vi "Set (Str).vi"(6 "ISOBUS address":T3=-1 caption="ISOBUS address (-1)", 8 "error in":errorcluster, 9 "Command Value (Str)":string, 10 "SCPI Message(s)":string[](array[string]), 11 "Mercury Reference In":T4) -> (0 "error out":errorcluster, 2 "Response":T1, 3 "Mercury Reference Out":T4, 4 "Valid?":T2)   [LabVIEW 2019]
doc: "Write the selected value as a string to the specified command on the remote instrument."
uses:
  Public/Controls/Mercury Reference.ctl
  Public/Controls/Comms Transport Layer.ctl
  Private/Controls/Query Dynamic Reference.ctl
  Public/Controls/ISOBus Address.ctl
  Public/Controls/Is Valid LED.ctl
  Public/Controls/Response String.ctl
  Mercury iXX.lvlib
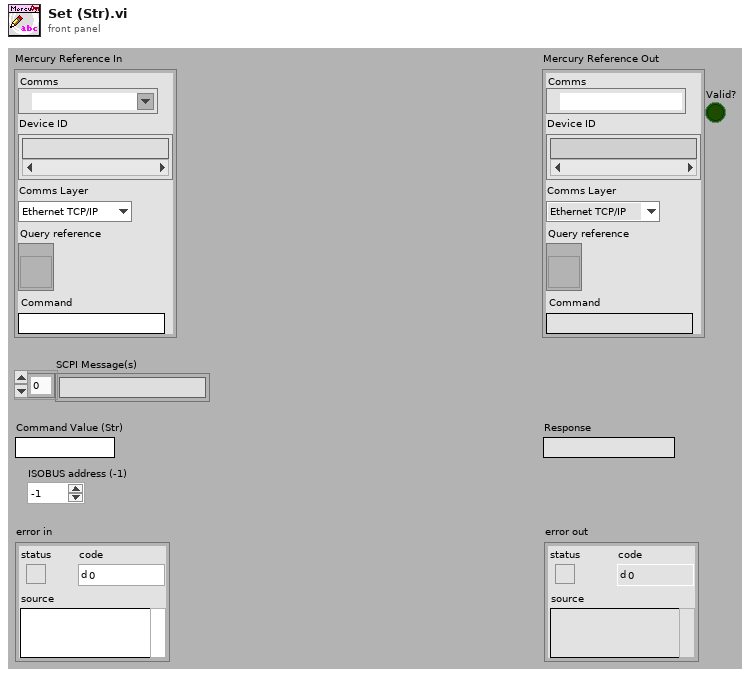
[diagram p1: front panel]
types:
  T1 = typedef "Mercury iXX.lvlib/Response String.ctl" = string
  T2 = typedef "Mercury iXX.lvlib/Is Valid LED.ctl" = bool
  T3 = typedef "Mercury iXX.lvlib/ISOBus Address.ctl" = i32
  T4 = typedef "Mercury iXX.lvlib/Mercury Reference.ctl" = cluster{"Comms":refnum<visa-resource-name>, "Device ID":string[], "Comms Layer":T5, "Command":string, "Query reference":T6}
  T5 = typedef "Mercury iXX.lvlib/Comms Transport Layer.ctl" = enum16{"Ethernet TCP/IP", "USB", "ISOBus - RS-232", "GPIB"}
  T6 = typedef "Mercury iXX.lvlib/Query Dynamic Reference.ctl" = refnum<vi>
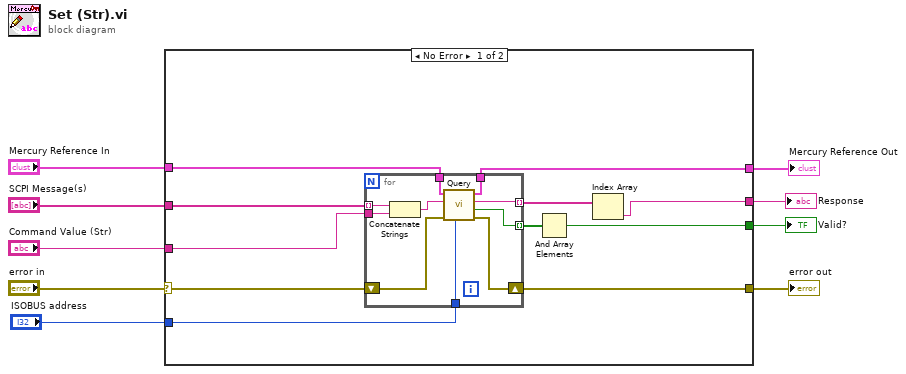
[diagram p0: block diagram]
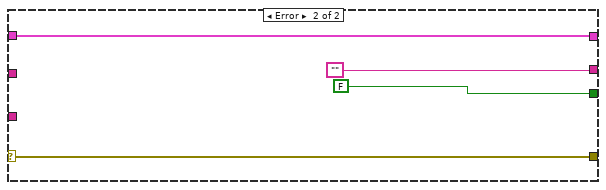
[diagram p2: hidden frame]
diagram:
  n1 = case shown="No Error" "error in" {
    selector: "error in" -> [w15 w33]
    tunnel: "Mercury Reference In" -> [w19 w34]
    tunnel: [w18 w34] -> w8
    tunnel: [w13 w33] -> w7
    tunnel: "ISOBUS address" -> [w14 _]
    tunnel: [w16 ""] -> w3
    tunnel: [w11 FALSE ("Valid?")] -> w4
    tunnel: "Command Value (Str)" -> [w20 _]
    tunnel: "SCPI Message(s)" -> [w10 _]
    frame No Error {
      n2 = for {
        tunnel: w10 -> [w30] mode=indexing
        tunnel: w20 -> [w29]
        tunnel: [w27] -> w17 mode=indexing
        tunnel: w19 -> [w26]
        tunnel: [w25] -> w18
        shift-right: [w23] -> w13
        shift-left: w15 -> [w24]
        tunnel: w14 -> [w22]
        tunnel: [w21] -> w12 mode=indexing
        n3 = Concatenate Strings(w30, w29) -> (w28:string)
        n4 = call "Query.vi"("ISOBUS address"=w22, "error in"=w24, "Command"=w28, "Mercury Reference In"=w26) -> ("error out"=w23:errorcluster, "Valid?"=w21:bool, "Data"=w27:string, "Mercury Reference Out"=w25:T4)  [unwired: 1 in, 3 out]
      }
      n5 = And Array Elements(Boolean array=w12) -> (logical AND=w11:bool)
      n6 = Index Array(array=w17) -> (element=w16:string)  [unwired: 1 in]
    }
    frame Error {
    }
  }
  "Mercury Reference Out" <- w8
  "error out" <- w7
  "Valid?" <- w4
  "Response" <- w3
